vi "Read_Axis_Position_tl.vi"(0 "Axis":string) -> (1 "Position":dbl format="%.2f", 2 "Index":i32)   [LabVIEW 2010]
doc: "Extracts the position of a given axis from the traverse global.\nAlso returns the index within the array aof given axis."
uses:
  Traverse_setup_tl.glob.vi
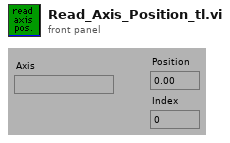
[diagram p1: front panel]
types:
  T1 = typedef "Axis_pos_cluster_tl.ctl" = cluster{"axis":string, "mac position":dbl}
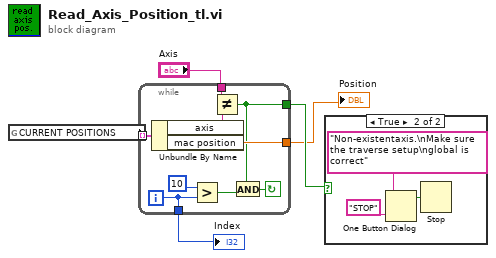
[diagram p0: block diagram]
diagram:
  n1 = global read "Traverse_setup_tl.glob.vi" "CURRENT POSITIONS"() -> (w5:T1[])
  n2 = while {
    tunnel: [w6] -> w1
    tunnel: [w7] -> w4
    tunnel: [w11] -> w2
    tunnel: "Axis" -> [w12]
    tunnel: w5 -> [w14] mode=indexing
    i -> [w6]
    stop <- w8 continue-if-true
    n3 = Unbundle By Name(w14) -> ("axis"=w13:string, "mac position"=w11:dbl)
    n4 = Greater?(x=10, y=w6) -> (0:w9:bool)
    n5 = Not Equal?(x=w12, y=w13) -> (x != y?=w7:bool)
    n6 = And(x=w7, y=w9) -> (x .and. y?=w8:bool)
  }
  "Position" <- w2
  "Index" <- w1
  n7 = case shown="True" w4 {
    frame False {
    }
    frame True {
      n8 = One Button Dialog(message="Non-existentaxis.\nMake sure the traverse setup\nglobal is correct", button name ("OK")="STOP") -> (true=w15:bool)
      n9 = Stop(stop? (T)=w15) -> ()
    }
  }
